vi "Write Sequence Name.vi"(8 "error in (no error)":errorcluster, 10 "Sequence Name":string, 11 "SequenceRepo in":refnum<class "SequenceRepo.lvclass">) -> (0 "error out":errorcluster, 3 "SequenceRepo out":refnum<class "SequenceRepo.lvclass">)   [LabVIEW 2015, in "SequenceRepo.lvclass"]
uses:
  SequenceRepo.lvclass
  SequenceRepo.lvclass/SequenceRepo.ctl
  Prototype/classes/Sequence/Config/Sequence Config.lvclass
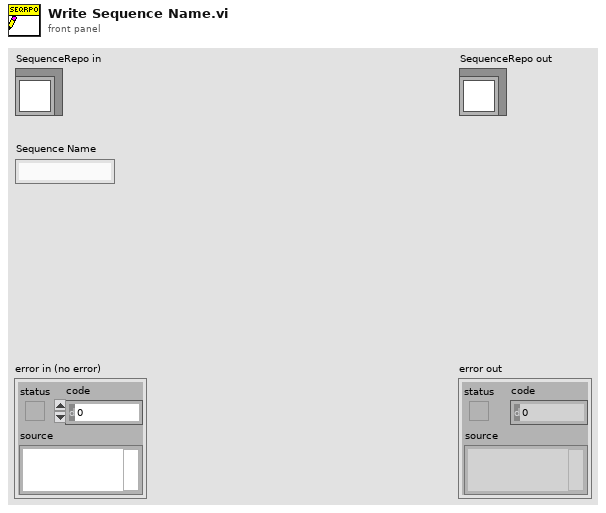
[diagram p1: front panel]
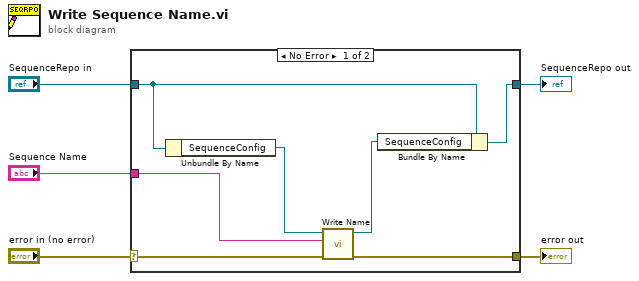
[diagram p0: block diagram]
diagram:
  n1 = case shown="No Error" "error in (no error)" {
    selector: "error in (no error)" -> [w7 w13]
    tunnel: [w6 w13] -> w4
    tunnel: [w8 w14] -> w2
    tunnel: "SequenceRepo in" -> [w9 w14]
    tunnel: "Sequence Name" -> [w10 _]
    frame No Error {
      n2 = Unbundle By Name(w9) -> ("SequenceConfig"=w12:refnum<class "Sequence Config.lvclass">)
      n3 = call-dynamic "Write Name.vi"("error in (no error)"=w7, "Name"=w10, "Sequence in"=w12) -> ("error out"=w6:errorcluster, "Sequence out"=w11:refnum<class "Sequence Config.lvclass">)  [unwired: 7 in]
      n4 = Bundle By Name(cluster=w9, "SequenceConfig"=w11) -> (w8:refnum<class "SequenceRepo.lvclass">)
    }
    frame Error {
    }
  }
  "error out" <- w4
  "SequenceRepo out" <- w2
